vi "FXP NILIA_OnePoleARM_IIR.vi"(1 "alpha [U16.0]":fxp<+,16,0>, 3 "x":fxp<+/-,18,3>) -> (0 "y[n]":fxp<+/-,32,3> format="%.30g")   [LabVIEW 2010]
uses:
  <vilib>/rvi/FXPMathLib/FxpMul/XNode/nifxpmath_Multiplier.xnode
  <vilib>/rvi/FXPMathLib/FxpMul/subVIs/nifxpmath_Mul_SimConfig.ctl
  <vilib>/fxp/LVFixedPointQuantizationPolicyTypeDef.ctl
  <vilib>/fxp/LVFixedPointOverflowPolicyTypeDef.ctl
  <vilib>/rvi/FXPMathLib/FxpAdd/XNode/nifxpmath_Add.xnode
  <vilib>/rvi/FXPMathLib/FxpAdd/subVIs/nifxpmath_Add_SimConfig.ctl
  <vilib>/rvi/FXPMathLib/FxpMul/simVIs/DllFxpMulTemp_sub.vi
  <vilib>/rvi/FXPMathLib/FxpAdd/simVIs/DllFxpAddTemp_sub.vi
panel:
  # "Pole location: 1-alpha\nH[z] = alpha/(1-z^-1 * (1-alpha))"
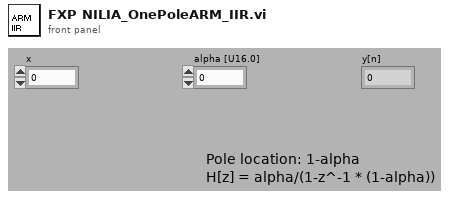
[diagram p1: front panel]
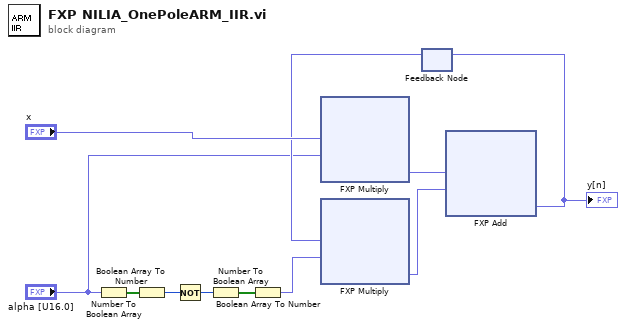
[diagram p0: block diagram]
diagram:
  n1 = Number To Boolean Array(number="alpha [U16.0]") -> (Boolean array=w7:bool[])
  n2 = Boolean Array To Number(Boolean array=w7) -> (number=w6:u16)
  n3 = Not(x=w6) -> (.not. x?=w5:u16)
  n4 = Number To Boolean Array(number=w5) -> (Boolean array=w4:bool[])
  n5 = Boolean Array To Number(Boolean array=w4) -> (number=w2:fxp<+,16,0>)
  n6 = xnode "FXP Multiply"("x"="x", "y"="alpha [U16.0]") -> ("x*y"=w10:fxp<+/-,32,3>)
  n7 = feedback #1() -> (w8:fxp<+/-,32,3>)  [unwired: 1 out]
  n8 = xnode "FXP Multiply"("x"=w8, "y"=w2) -> ("x*y"=w1:fxp<+/-,32,3>)
  n9 = xnode "FXP Add"("x"=w10, "y"=w1) -> ("x+y"=w9:fxp<+/-,32,3>)
  "y[n]" <- w9
  n10 = feedback-in #1(w9) -> ()
